vi "DélaisGen.vi"(8 "error in (no error)":errorcluster caption="entrée d'erreur", 11 "Numérique":u32) -> (0 "error out":errorcluster caption="sortie d'erreur")   [LabVIEW 2010]
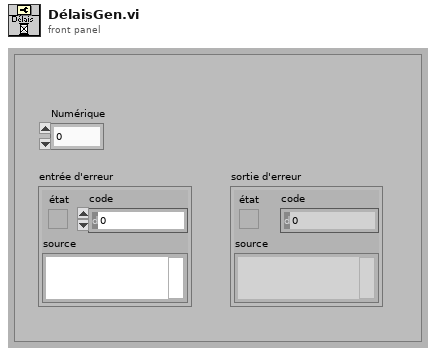
[diagram p1: front panel]
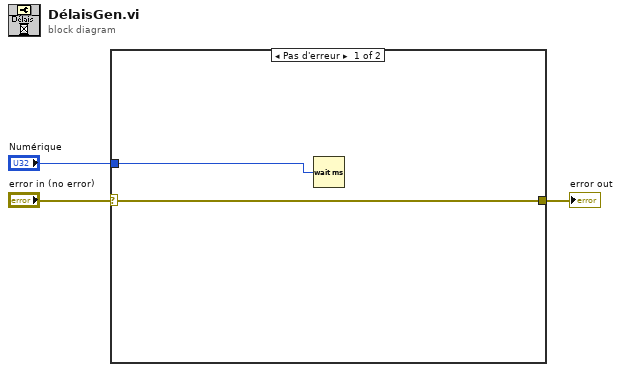
[diagram p0: block diagram]
diagram:
  n1 = case shown="Pas d'erreur" "error in (no error)" {
    selector: "error in (no error)" -> [w5 w6]
    tunnel: "Numérique" -> [w4 _]
    tunnel: [w5 w6] -> w1
    frame No Error {
      n2 = Wait (ms)(milliseconds to wait=w4) -> ()  [unwired: 1 out]
    }
    frame Error {
    }
  }
  "error out" <- w1
